vi "COVSubVI.vi"(1 "Array":dbl[][](array[numeric])) -> (0 "Numeric":dbl)   [LabVIEW 2021]
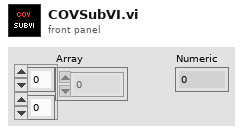
[diagram p1: front panel]
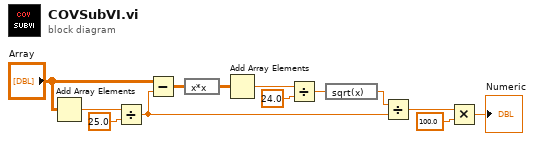
[diagram p0: block diagram]
diagram:
  n1 = Add Array Elements(numeric array="Array") -> (sum=w1:dbl)
  n2 = Divide(x=w1, y=25.0) -> (x/y=w8:dbl)
  n3 = Subtract(x="Array", y=w8) -> (x-y=w4:dbl[][])
  n4 = expression code="x*x"(w4) -> (w5:dbl[][])
  n5 = Add Array Elements(numeric array=w5) -> (sum=w6:dbl)
  n6 = Divide(x=w6, y=24.0) -> (x/y=w9:dbl)
  n7 = expression code="sqrt(x)"(w9) -> (w10:dbl)
  n8 = Divide(x=w10, y=w8) -> (x/y=w11:dbl)
  n9 = Multiply(x=w11, y=100.0) -> (x*y=→"Numeric":dbl)
